vi "Write Spreadsheet File.vi"(6 "Delimiter (tab)":string="\t", 8 "error in (no error)":errorcluster, 9 "Append to File? (F)":bool, 10 "2D String[][]":string[][](array[string]), 11 "File Path":path) -> (0 "error out":errorcluster, 3 "File Path dup":path)   [LabVIEW 2014, in "SLL Spreadsheet.lvlib"]
doc: "Supports writing of 2D string with new line & comma to a spreadsheet file, which are not supported by LabVIEW's builtin function.\n\nIts functionality is similar to how Excel does it - it adds double quotes to cells which contains new line character, comma and double quotes. If the cell already has double quotes, it escapes it with one more double quotes."
uses:
  SLL Spreadsheet.lvlib
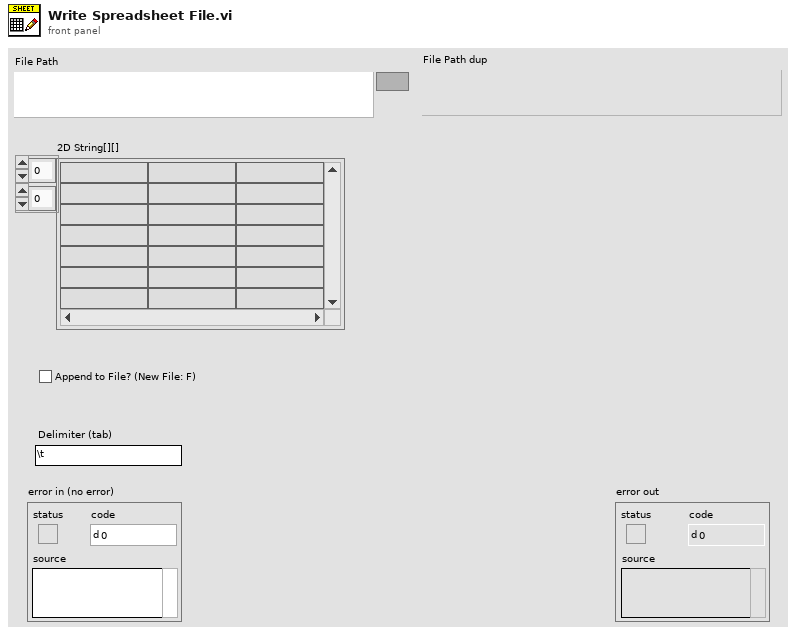
[diagram p1: front panel]
types:
  T1 = enum16{"open", "replace", "create", "open or create", "replace or create", "replace or create with confirmation"}
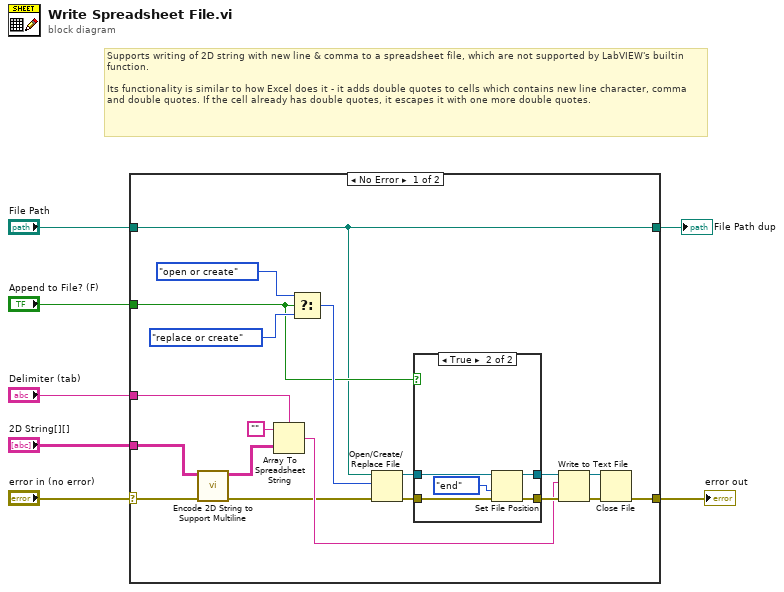
[diagram p0: block diagram]
diagram:
  # "Supports writing of 2D string with new line & comma to a spreadsheet file, which are not supported by LabVIEW's builtin function.\n\nIts functionality is similar to how Excel does it - it adds double quotes to cells which contains new line character, comma and double quotes. If the cell already has double quotes, it escapes it with one more double quotes."
  n1 = case shown="No Error" "error in (no error)" {
    selector: "error in (no error)" -> [w10 w35]
    tunnel: "Append to File? (F)" -> [w17 _]
    tunnel: [w16 w35] -> w6
    tunnel: "2D String[][]" -> [w15 _]
    tunnel: "Delimiter (tab)" -> [w13 _]
    tunnel: "File Path" -> [w8 w34]
    tunnel: [w8 w34] -> w1
    frame No Error {
      n2 = call "Encode 2D String to Support Multiline.vi"("error in (no error)"=w10, "2D Array In"=w15) -> ("error out"=w9:errorcluster, "2D Array Out"=w14:string[][])  [unwired: 8 in]
      n3 = Array To Spreadsheet String(delimiter (Tab)=w13, array=w14, 3:"") -> (spreadsheet string=w12:string)
      n4 = Select ("function")(t=T1."open or create" ("operation (0:open)"), s=w17, f=T1."replace or create" ("operation (0:open)")) -> (s? t:f=w22:T1)
      n5 = Open/Create/Replace File(file path (use dialog)=w8, error in=w9, operation (0:open)=w22) -> (refnum out=w19:refnum<file>, error out=w20:errorcluster)  [unwired: 3 in, 1 out]
      n6 = case shown="True" w17 {
        tunnel: w20 -> [w27 w33]
        tunnel: [w27 w32] -> w21
        tunnel: w19 -> [w28 w30]
        tunnel: [w28 w31] -> w18
        frame False {
        }
        frame True {
          n7 = Set File Position(refnum=w30, from (0:start)=enum16{"start", "end", "current"}."end", error in=w33) -> (refnum out=w31:refnum<file>, error out=w32:errorcluster)  [unwired: 1 in]
        }
      }
      n8 = Write to Text File(file (use dialog)=w18, text=w12, error in=w21) -> (refnum out=w24:refnum<file>, error out=w23:errorcluster)  [unwired: 1 in, 1 out]
      n9 = Close File(refnum=w24, error in=w23) -> (error out=w16:errorcluster)  [unwired: 1 out]
    }
    frame Error {
    }
  }
  "error out" <- w6
  "File Path dup" <- w1
